vi "coupled mirror calibration.vi"(4 "seperation":dbl, 6 "distance to target plane":dbl, 7 "pixel calib":dbl, 8 "xCal 2":dbl, 9 "xCal":dbl, 10 "x'":dbl, 11 "x":dbl) -> (2 "A2x":dbl, 3 "A1x":dbl)   [LabVIEW 2020]
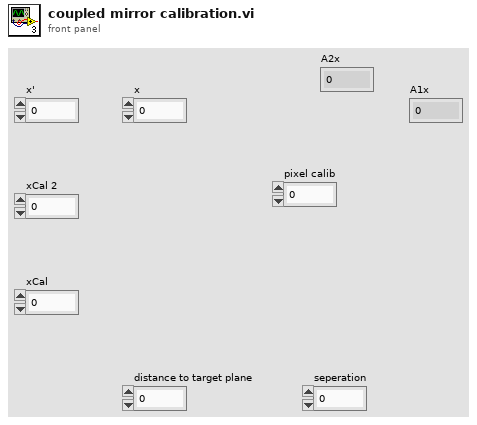
[diagram p1: front panel]
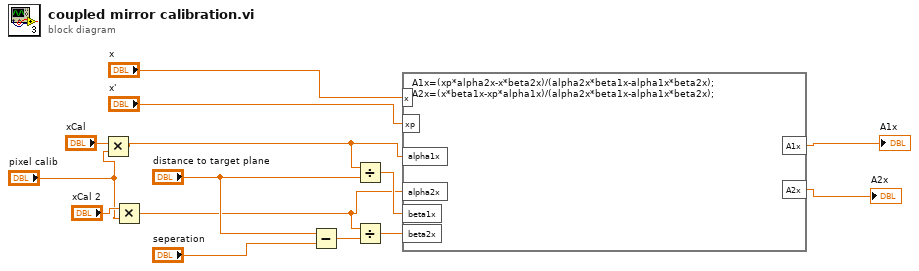
[diagram p0: block diagram]
diagram:
  n1 = Multiply(x="xCal", y="pixel calib") -> (x*y=w4:dbl)
  n2 = Multiply(x="xCal 2", y="pixel calib") -> (x*y=w1:dbl)
  n3 = Subtract(x="distance to target plane", y="seperation") -> (x-y=w12:dbl)
  n4 = Divide(x=w4, y="distance to target plane") -> (x/y=w10:dbl)
  n5 = Divide(x=w1, y=w12) -> (x/y=w11:dbl)
  n6 = formula code="A1x=(xp*alpha2x-x*beta2x)/(alpha2x*beta1x-alpha1x*beta2x);\nA2x=(x*beta1x-xp*alpha1x)/(alpha2x*beta1x-alpha1x*beta2x);"("x"="x", "xp"="x'", "alpha1x"=w4, "alpha2x"=w1, "beta1x"=w10, "beta2x"=w11) -> ("A1x"=→"A1x":dbl, "A2x"=→"A2x":dbl)
